vi "Channel_Identify.vi"(0 "Current Frequency Index":i32, 1 "Samples Before Measuring":i32[](array[numeric]), 2 "Current Sample":i32, 3 "In Frequency Sinusoids":cluster{"cos(wt)":dbl, " sin(wt)":dbl}, 4 "Samples for Calculation":i32[](array[numeric]), 5 "Frequency Response":dbl) -> (6 "Initalize":bool, 7 "Frequency Response Magnitude":dbl, 8 "Frequency Response  Phase":dbl)   [LabVIEW 2017]
doc: "Over a given number of cycles, calculates the magnitude and phase of a sinusoid at a given frequency.\n\nTo calculate the magnitude and phase of a sinusoid at a given frequency, the following steps are taken:\n\n 1.) The input sinusoid is multiplied by a sine wave and cosine wave at the same frequency:\n\n A*sin(wt+phi)*cos(wt) = 0.5*A*{ sin(phi) + sin(wt+phi) }\n A*sin(wt+phi)*sin(wt) = 0.5*A*{ cos(phi) - cos(wt+phi) }\n\n 2.) These two product waves are averaged over an inputted multiple of their period:\n\n MEAN{ A*sin(wt+phi)*cos(wt) } = 0.5*A*sin(phi)\n MEAN{ A*sin(wt+phi)*sin(wt) } = 0.5*A*cos(phi)\n\n 3.) The magnitude of the input sinusoid is found:\n\n Mag = 2*sqrt{ (0.5*A*sin(phi)^2 + (0.5*A*sin(phi)^2 } \n = 2*sqrt{ (0.5*A)^2 * (sin(phi)^2 + cos(phi)^2) }\n = 2* sqrt{ (0.5*A)^2 * 1} \n = 2*0.5*A\n = A\n\n 4.) Phase Detection\n\n Phase = arctan{ 0.5*A*sin(phi) / 0.5*A*cos(phi) }\n = arctan{ sin(phi) / cos(phi) } = arctan{ tan(phi) }\n = phi\n\n NOTE: atan2 is used of atan since it keeps track of quadrant for the arctan function.\n\nInputs: \n\n- Samples Before Measuring: A list of the last sample to be ignored for a given frequency. Following this sample, measuring should begin for a particular frequency.\n\n- Current Frequency Index: The index of the frequency which the frequency response (sinusoid) entered has.\n\n- Current Sample: The current sample being measured of the excited system. \n NOTE: Since we must excite the system before recording data, this will be the number of iterations the loop containing this function has run minus one.\n\n- In Frequency Sinusoids: A sine and cosine wave at the current excitation's frequency used to demodulate the system's frequency response to pull out the phase and magnitude.\n\n- Frequency Response: The sinusoid response of the system to the DSA's output excitation at the previous time step.\n\n- Samples for Calculation: A list of the number of samples to be measured per frequency to measure the frequency response.\n\nOutputs: \n\n- Intalize: Outputs TRUE if the sample beinging measured is the first sample measured for a new frequency to indicate the mean subvi within this vi has be restarted.\n\n- Frequency Response Magnitude: The magnitude of the frequncy response input. \n NOTE: This value is only accurate once this vi has averaged all the number of input samples of the frequency response for a given amount of full cycles.\n\n- Frequency Response Phase: The phase of the frequncy response input. \n NOTE: This value is only accurate once this vi has averaged all the number of input samples of the frequency response for a given amount of full cycles."
uses:
  <vilib>/ptbypt/NI_PtbyPt.lvlib
panel:
  # "Channel_Identify"
  # "Indentication Inputs"
  # "Indentication Outputs"
  # "Measurement Properties"
  # "Frequency Response Components"
  # "Phase"
  # "Magnitude"
  # "Per Frequency"
  # "Measuring"
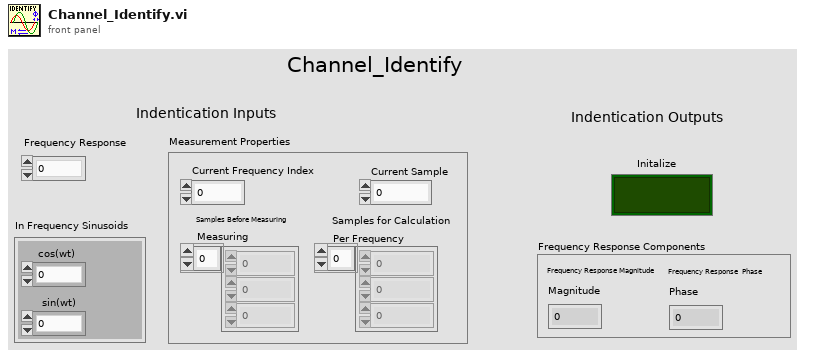
[diagram p1: front panel]
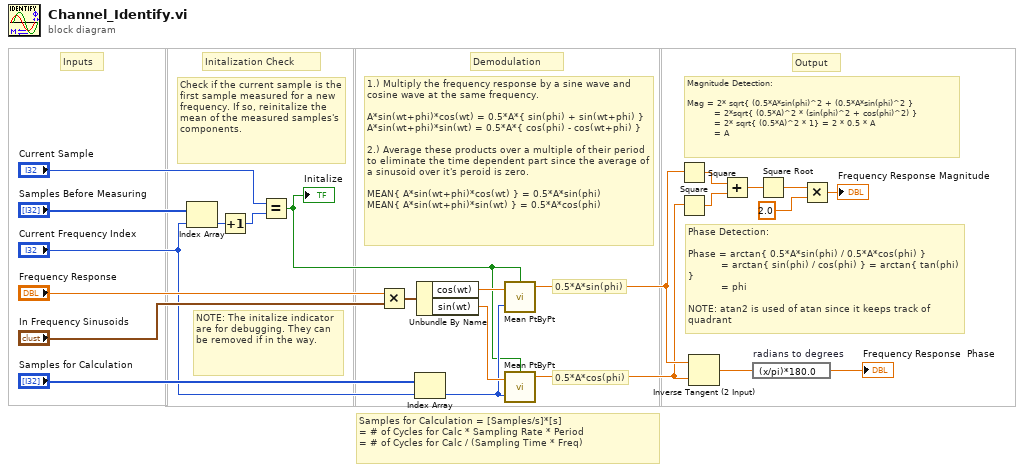
[diagram p0: block diagram]
diagram:
  # "NOTE: The initalize indicator are for debugging. They can be removed if in the way."
  # "0.5*A*cos(phi)"
  # "0.5*A*sin(phi)"
  # "Phase Detection:\n\nPhase = arctan{ 0.5*A*sin(phi) / 0.5*A*cos(phi) }\n           = arctan{ sin(phi) / cos(phi) } = arctan{ tan(phi) }\n           = phi\n\nNOTE: atan2 is used of atan since it keeps track of quadrant"
  # "Magnitude Detection:\n\nMag = 2* sqrt{ (0.5*A*sin(phi)^2 + (0.5*A*sin(phi)^2 } \n         = 2*sqrt{ (0.5*A)^2 * (sin(phi)^2 + cos(phi)^2) }\n         = 2* sqrt{ (0.5*A)^2 * 1} = 2 * 0.5 * A\n         = A"
  # "Output"
  # "Samples for Calculation = [Samples/s]*[s]\n= # of Cycles for Calc * Sampling Rate * Period\n= # of Cycles for Calc / (Sampling Time * Freq)"
  # "1.) Multiply the frequency response by a sine wave and cosine wave at the same frequency.\n\nA*sin(wt+phi)*cos(wt) = 0.5*A*{ sin(phi) + sin(wt+phi) }\nA*sin(wt+phi)*sin(wt) = 0.5*A*{ cos(phi) - cos(wt+phi) }\n\n2.) Average these products over a multiple of their period to eliminate the time dependent part since the average of a sinusoid over it's peroid is zero. \n\nMEAN{ A*sin(wt+phi)*cos(wt) } = 0.5*A*sin(phi)\nMEAN{ A*sin(wt+phi)*sin(wt) } = 0.5*A*cos(phi)"
  # "Demodulation"
  # "Check if the current sample is the first sample measured for a new frequency. If so, reinitalize the mean of the measured samples's components."
  # "Initalization Check"
  # "Inputs"
  n1 = Index Array(array="Samples Before Measuring", index="Current Frequency Index") -> (element=w22:i32)
  n2 = Increment(x=w22) -> (x+1=w21:i32)
  n3 = Equal?(x="Current Sample", y=w21) -> (x = y?=w11:bool)
  "Initalize" <- w11
  n4 = Multiply(x="Frequency Response", y="In Frequency Sinusoids") -> (x*y=w17:cluster{"cos(wt)":dbl, " sin(wt)":dbl})
  n5 = Index Array(array="Samples for Calculation", index="Current Frequency Index") -> (element=w12:i32)
  n6 = Unbundle By Name(w17) -> ("cos(wt)"=w14:dbl, "sin(wt)"=w13:dbl)
  n7 = call <vilib>:"Mean PtByPt.vi"("x"=w14, "sample length"=w12, "initialize"=w11) -> ("mean"=w5:dbl)  [unwired: 1 in, 1 out]
  n8 = call <vilib>:"Mean PtByPt.vi"("x"=w13, "sample length"=w12, "initialize"=w11) -> ("mean"=w4:dbl)  [unwired: 1 in, 1 out]
  n9 = Square(x=w5) -> (x^2=w10:dbl)
  n10 = Square ("Square 2")(x=w4) -> (x^2=w9:dbl)
  n11 = Inverse Tangent (2 Input)(1:w4, 2:w5) -> (0:w3:dbl)
  n12 = Add(x=w10, y=w9) -> (x+y=w8:dbl)
  n13 = expression code="(x/pi)*180.0" "radians to degrees"(w3) -> (→"Frequency Response  Phase":dbl)
  n14 = Square Root(x=w8) -> (sqrt(x)=w7:dbl)
  n15 = Multiply ("Multiply 3")(x=w7, y=2.0) -> (x*y=→"Frequency Response Magnitude":dbl)
